vi "Write.vi"(8 "error in (no error)":errorcluster, 10 "Data":string, 11 "DeployResource in":refnum<class "Resource.lvclass">) -> (0 "error out":errorcluster, 3 "DeployResource out":refnum<class "Resource.lvclass">)   [LabVIEW 2020, in "PicoG-Core.lvlib" / "Resource.lvclass"]
uses:
  Resource.lvclass
  Resource.lvclass/Resource.ctl
  <vilib>/IlluminatedG/lv-stream/stream/Stream.lvclass
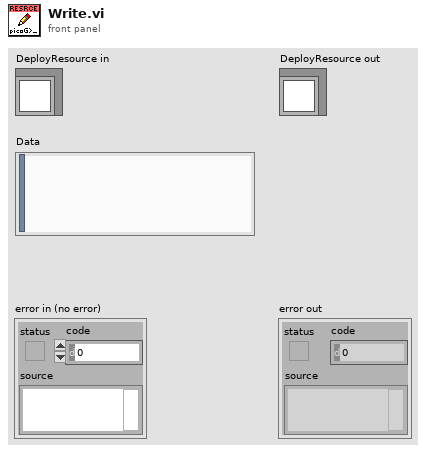
[diagram p1: front panel]
types:
  T1 = typedef "PicoG-Core.lvlib/Resource.lvclass/Ref Data.ctl" = cluster{"Config":map{string, string}, "Client":refnum<class "Connection.lvclass">, "Stream":refnum<class "Stream.lvclass">}
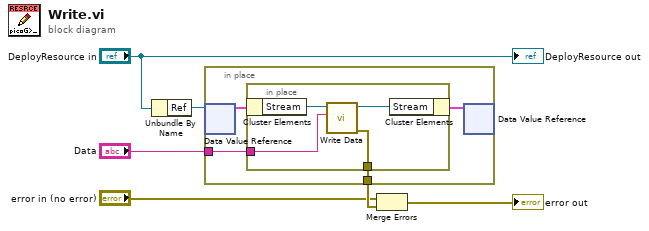
[diagram p0: block diagram]
diagram:
  n1 = Unbundle By Name("DeployResource in") -> ("Ref"=w6:refnum<data-value>)
  n2 = in-place {
    in-place-border: "Data" -> [w8]
    in-place-border: [w7] -> w3
    n3 = in-place-dvr #1(w6) -> (w10:T1)  [unwired: 1 out]
    n4 = in-place {
      in-place-border: w8 -> [w12]
      in-place-border: [w11] -> w7
      n5 = in-place-cluster #2(w10) -> ("Stream"=w14:refnum<class "Stream.lvclass">)
      n6 = call <vilib>:"Write Data.vi"("Data"=w12, "Stream in"=w14) -> ("error out"=w11:errorcluster, "Stream out"=w13:refnum<class "Stream.lvclass">)  [unwired: 8 in]
      n7 = in-place-cluster #2("Stream"=w13) -> (w9:T1)
    }
    n8 = in-place-dvr #1(w9) -> ()  [unwired: 2 out]
  }
  n9 = Merge Errors("error in (no error)", w3) -> (→"error out":errorcluster)
  "DeployResource out" <- "DeployResource in"
